vi "Convert From Tree To Element.vi"(8 "error in":errorcluster, 11 "Tree in":refnum<class "Tree.lvclass">) -> (0 "error out":errorcluster, 2 "ELEMENT":T1, 3 "Tree out":refnum<class "Tree.lvclass">)   [LabVIEW 2019]
uses:
  Tree/Tree.lvclass
  DataTypes/Base/GDSII.DataType.lvclass
  TypeDefs/ELEMENT.ctl
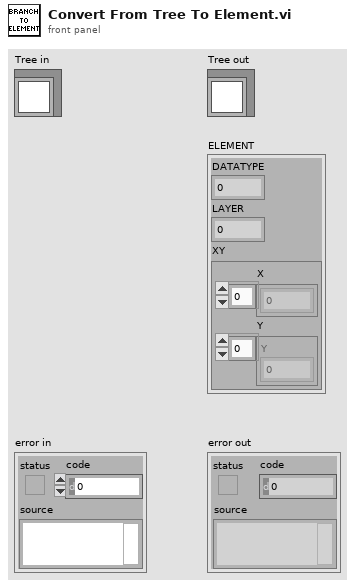
[diagram p1: front panel]
types:
  T1 = typedef "ELEMENT.ctl" = cluster{"DATATYPE":i16, "LAYER":i16, "XY":cluster{"X":i32[], "Y":i32[]}}
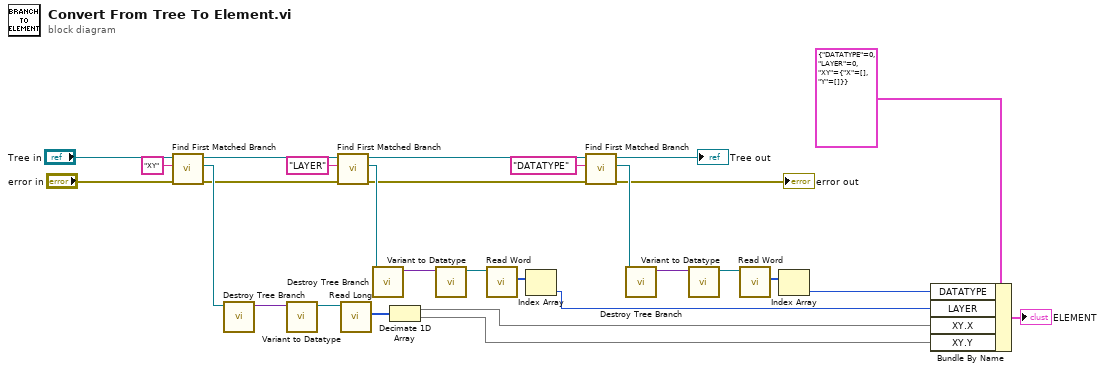
[diagram p0: block diagram]
diagram:
  n1 = call "Find First Matched Branch.vi"("error in"="error in", "Branch Name Exact"="XY", "Tree in"="Tree in") -> ("error out"=w21:errorcluster, "Matched Branch"=w27:refnum<class "Tree.lvclass">, "Tree out"=w23:refnum<class "Tree.lvclass">)  [unwired: 5 in, 1 out]
  n2 = call "Destroy Tree Branch.vi"("Tree in"=w27) -> ("Root"=w26:variant)  [unwired: 9 in, 1 out]
  n3 = call "Variant to Datatype.vi"("Variant"=w26) -> ("DataType"=w25:refnum<class "GDSII.DataType.lvclass">)  [unwired: 9 in, 1 out]
  n4 = call "Find First Matched Branch.vi"("error in"=w21, "Branch Name Exact"="LAYER", "Tree in"=w23) -> ("error out"=w14:errorcluster, "Matched Branch"=w19:refnum<class "Tree.lvclass">, "Tree out"=w15:refnum<class "Tree.lvclass">)  [unwired: 5 in, 1 out]
  n5 = call-dynamic "Read Long.vi"("GDSII.DataType in"=w25) -> ("Long"=w24:i32[])  [unwired: 9 in, 1 out]
  n6 = call "Destroy Tree Branch.vi"("Tree in"=w19) -> ("Root"=w20:variant)  [unwired: 9 in, 1 out]
  n7 = Decimate 1D Array(w24) -> (w3:i32[], w2:i32[])
  n8 = call "Variant to Datatype.vi"("Variant"=w20) -> ("DataType"=w18:refnum<class "GDSII.DataType.lvclass">)  [unwired: 9 in, 1 out]
  n9 = call-dynamic "Read Word.vi"("GDSII.DataType in"=w18) -> ("Word"=w17:i16[])  [unwired: 9 in, 1 out]
  n10 = Index Array(array=w17) -> (element=w4:i16)  [unwired: 1 in]
  n11 = call "Find First Matched Branch.vi"("error in"=w14, "Branch Name Exact"="DATATYPE", "Tree in"=w15) -> ("error out"=→"error out":errorcluster, "Matched Branch"=w10:refnum<class "Tree.lvclass">, "Tree out"=→"Tree out":refnum<class "Tree.lvclass">)  [unwired: 5 in, 1 out]
  n12 = call "Destroy Tree Branch.vi"("Tree in"=w10) -> ("Root"=w11:variant)  [unwired: 9 in, 1 out]
  n13 = call "Variant to Datatype.vi"("Variant"=w11) -> ("DataType"=w12:refnum<class "GDSII.DataType.lvclass">)  [unwired: 9 in, 1 out]
  n14 = call-dynamic "Read Word.vi"("GDSII.DataType in"=w12) -> ("Word"=w13:i16[])  [unwired: 9 in, 1 out]
  n15 = Index Array(array=w13) -> (element=w5:i16)  [unwired: 1 in]
  n16 = Bundle By Name(cluster=T1 {"DATATYPE"=0, "LAYER"=0, "XY"={"X"=[], "Y"=[]}} ("ELEMENT"), "DATATYPE"=w5, "LAYER"=w4, "XY.X"=w3, "XY.Y"=w2) -> (→"ELEMENT":T1)
